vi "Update Dynamic Shunt Default Values.vi"(8 "error in (no error)":errorcluster, 9 "Dynamic shunt?":bool, 10 "9235 in":refnum<class "9235.lvclass">, 11 "Node Ptr in":T1 format="%.0x") -> (0 "error out":errorcluster, 2 "9235 out":refnum<class "9235.lvclass">, 3 "Node Ptr out":T1 format="%.0x")   [LabVIEW 2017, in "Modules.lvlib" / "9235.lvclass"]
uses:
  9235.lvclass
  <vilib>/NI Veristand/Custom Device API/Custom Device Item Ref.ctl
  9235.lvclass/9235.ctl
  RSI Module/Channel GUIDs.vi
  <vilib>/NI Veristand/Custom Device Tools/Custom Device Utility Library/NI VeriStand - Search for Item by GUID.vi
  <vilib>/NI Veristand/Custom Device Tools/Custom Device Utility Library/Custom Device Utility Library.lvlib
  RSI Module/RSI Module.lvclass
  <vilib>/NI Veristand/Custom Device API/Custom Device API.lvlib
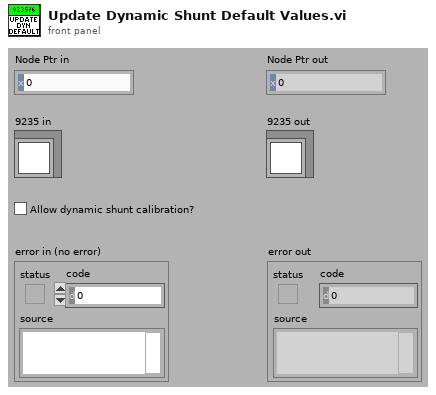
[diagram p1: front panel]
types:
  T1 = typedef "Custom Device API.lvlib/Custom Device Item Ref.ctl" = u64
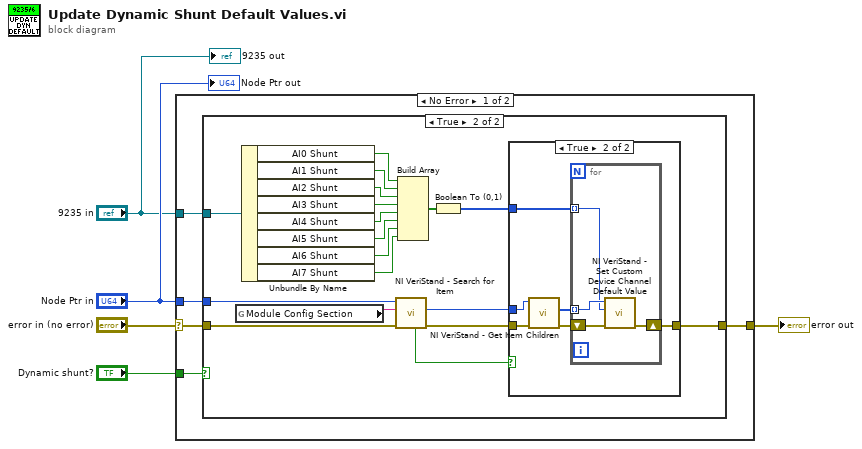
[diagram p0: block diagram]
diagram:
  n1 = case shown="No Error" "error in (no error)" {
    selector: "error in (no error)" -> [w7 w41]
    tunnel: [w6 w41] -> w4
    tunnel: "9235 in" -> [w9 _]
    tunnel: "Dynamic shunt?" -> [w10 _]
    tunnel: "Node Ptr in" -> [w8 _]
    frame No Error {
      n2 = case shown="True" w10 {
        tunnel: w9 -> [_ w13]
        tunnel: w8 -> [_ w25]
        tunnel: w7 -> [w11 w24]
        tunnel: [w11 w23] -> w6
        frame False {
        }
        frame True {
          n3 = global read "Channel GUIDs.vi" "Module Config Section"() -> (w29:string)
          n4 = Unbundle By Name(w13) -> ("AI0 Shunt"=w22:bool, "AI1 Shunt"=w21:bool, "AI2 Shunt"=w20:bool, "AI3 Shunt"=w19:bool, "AI4 Shunt"=w17:bool, "AI5 Shunt"=w16:bool, "AI6 Shunt"=w15:bool, "AI7 Shunt"=w14:bool)
          n5 = call-poly <vilib>:"NI VeriStand - Search for Item.vi"("error in"=w24, "Item GUID"=w29, "Section Ref in"=w25) -> ("error out"=w27:errorcluster, "Item Ref"=w26:T1, "Found"=w28:bool)  [unwired: 5 in, 1 out]
          n6 = Build Array(w22, w21, w20, w19, w17, w16, w15, w14) -> (w18:bool[])
          n7 = Boolean To (0,1)(Boolean=w18) -> (0, 1=w12:i16[])
          n8 = case shown="True" w28 {
            tunnel: w27 -> [w30 w36]
            tunnel: w26 -> [_ w35]
            tunnel: [w30 w33] -> w23
            tunnel: w12 -> [_ w31]
            frame False {
            }
            frame True {
              n9 = call <vilib>:"NI VeriStand - Get Item Children.vi"("error in (no error)"=w36, "Item Ref in"=w35) -> ("error out"=w34:errorcluster, "Child Refs"=w32:T1[])  [unwired: 6 in, 2 out]
              n10 = for {
                shift-right: [w39] -> w33
                shift-left: w34 -> [w40]
                tunnel: w32 -> [w38] mode=indexing
                tunnel: w31 -> [w37] mode=indexing
                n11 = call <vilib>:"NI VeriStand - Set Custom Device Channel Default Value.vi"("error in (no error)"=w40, "Default Value"=w37, "Channel Ref in"=w38) -> ("error out"=w39:errorcluster)  [unwired: 7 in, 1 out]
              }
            }
          }
        }
      }
    }
    frame Error {
    }
  }
  "error out" <- w4
  "9235 out" <- "9235 in"
  "Node Ptr out" <- "Node Ptr in"
